vi "Synchronized AO Generation.vi"() -> ()   [LabVIEW 2018, in "GettingStarted_5785_Host.lvlib"]
uses:
  GettingStarted_5785_Host.lvlib
  <vilib>/userdefined/High Color/nirio_resource_hc.ctl
  <instrlib>/FlexRIO/API/Host/v1/NI FlexRIO/API/Get Property Reference - Fpga Small.vi
  <instrlib>/FlexRIO/API/Host/v1/NI FlexRIO/API/Configure Digital Edge Start Trigger.vi
  <instrlib>/FlexRIO/API/Host/v1/NI FlexRIO/API/Read Stream 1D WDT.vi
  <vilib>/FPGAPlugInAG/Dynamic/niLvFpga_Close_Dynamic.vi
  <vilib>/rvi/interface/nirviCloseFPGA/nirviCloseFPGA.xnode
  <resource>/objmgr/niflexrioapiStream.rc
  <instrlib>/FlexRIO/API/Host/v1/NI FlexRIO API v1.lvlib
  <resource>/objmgr/niflexrioapi.rc
  <instrlib>/_niInstr/Streaming/v1/Host/niInstr Streaming v1 Host.lvlib
panel:
  in  "flexrio tranceivers":T2(array[cluster])
  in  "amplitude":dbl=0.2 format="%0.2p"
  in  "sampling info":cluster{"Fs":dbl, "#s":dbl}={"Fs"=3200000000.0, "#s"=1600.0} {"Fs" format="%#_6p"}
  in  "frequency":dbl=32000000.0 format="%0.2p"
  out "read data":waveform(dbl)[](graph)
  in  "num samples":u64=65536
  out "generation active":bool[](array[boolean])
  in  "stop":bool
  in  "trigger source":string(combo)
  in  "trigger mode":enum16{"Immediate", "Digital"}(ring)
  out "error out":errorcluster
  # "This example demonstrates how to synchronize AO streams across multiple transceivers.\n\nThe same waveform is downloaded to each each device, and generation will begin on AO0 and AO1 when the start trigger is received.\n\nChannels AI0 and AI1 on the first device are continually acquired and displayed.\n\nThe suggested cable configuration is to loopback AO0 to AI0 on the first device, and connect AO0 from the second device to AI1 on the first device."
  # "Generation trigger configuration"
  # "Digital Trigger configuration"
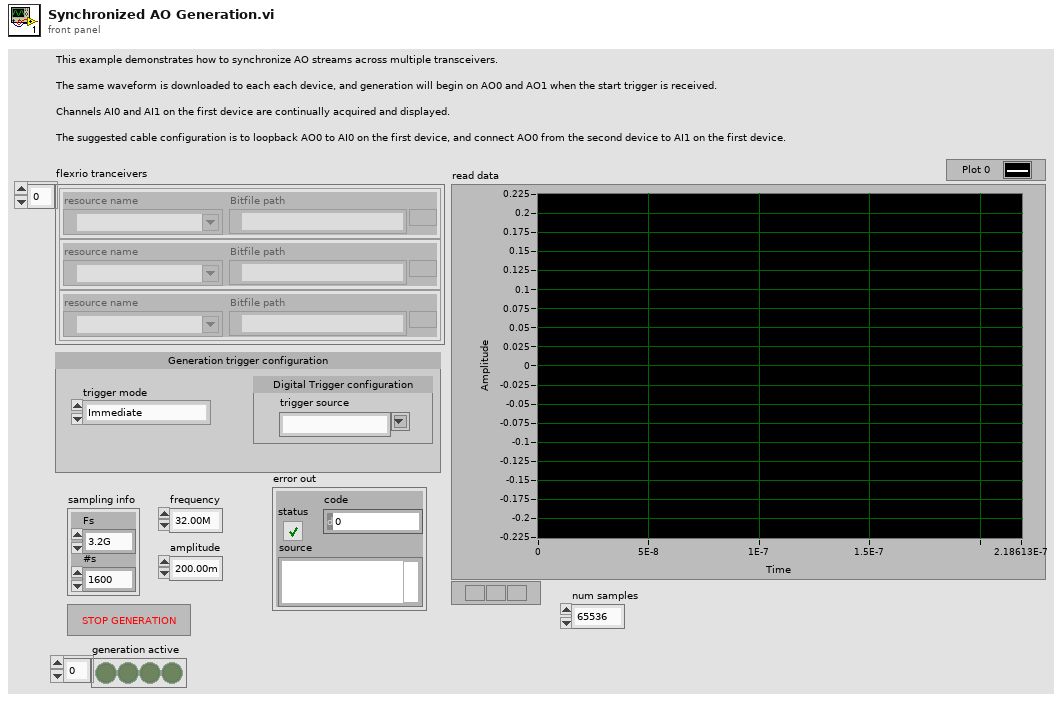
[diagram p1: front panel]
types:
  T1 = typedef "nirio_resource_hc.ctl" = tag
  T2 = cluster{"resource name":T1, "Bitfile path":path}[]
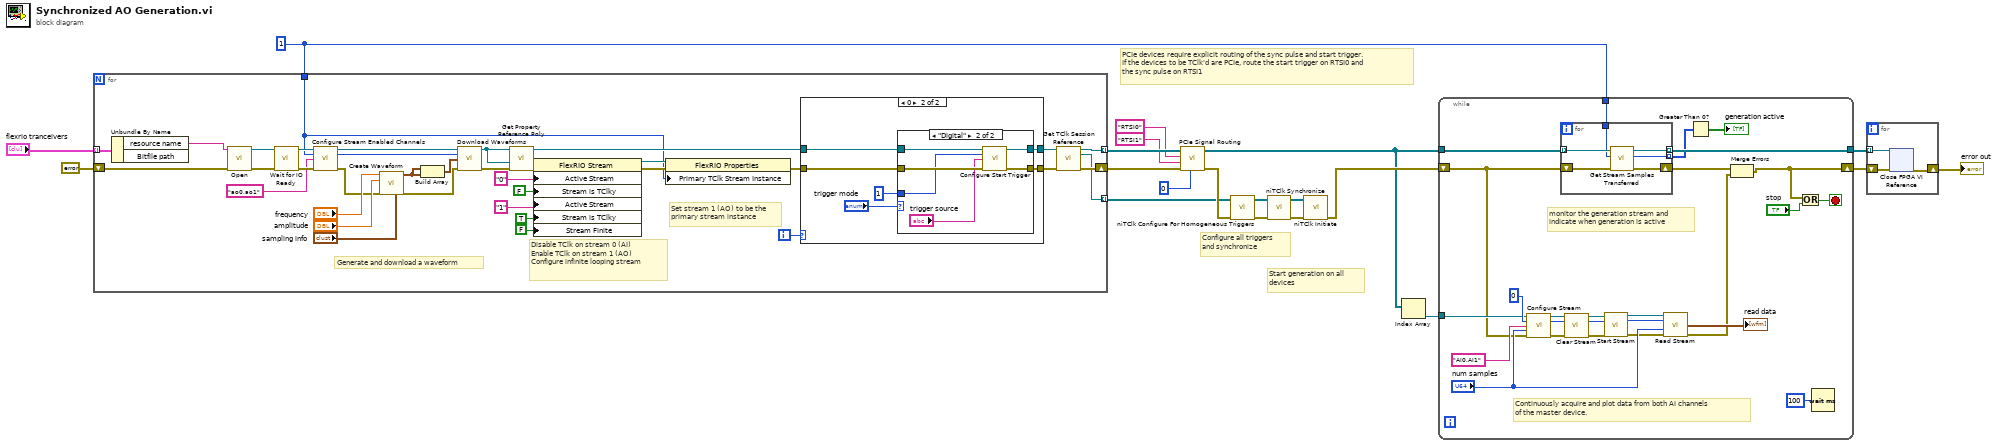
[diagram p0: block diagram]
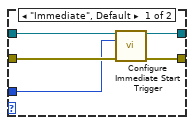
[diagram p3: hidden frame]
diagram:
  w3 = u32 1 ("stream instance")
  # "PCIe devices require explicit routing of the sync pulse and start trigger.\nIf the devices to be TClk'd are PCIe, route the start trigger on RTSI0 and\nthe sync pulse on RTSI1"
  # "Configure all triggers \nand synchronize"
  # "Start generation on all devices"
  n1 = for {
    tunnel: "flexrio tranceivers" -> [w40] mode=indexing
    tunnel: [w33] -> w7 mode=indexing
    shift-right: [w32] -> w9
    shift-left: errorcluster {"status"=FALSE, "code"=0, "source"=""} ("error out") -> [w48]
    tunnel: [w31] -> w6 mode=indexing
    tunnel: w3 -> [w23]
    i -> [w29]
    # "Set stream 1 (AO) to be the\nprimary stream instance"
    # "Disable TClk on stream 0 (AI)\nEnable TClk on stream 1 (AO)\nConfigure infinite looping stream"
    # "Generate and download a waveform"
    n2 = Unbundle By Name(w40) -> ("resource name"=w39:T1)  [unwired: 1 out]
    n3 = call <instrlib>:"Open.vi"("RIO Device"=w39, "error in"=w48) -> ("fpga interface out"=w37:refnum<k20>, "error out"=w38:errorcluster)  [unwired: 12 in]
    n4 = call <instrlib>:"Wait for IO Ready.vi"("fpga interface in"=w37, "error in"=w38) -> ("fpga interface out"=w27:refnum<k20>, "error out"=w26:errorcluster)  [unwired: 10 in, 2 out]
    n5 = call <instrlib>:"Configure Stream Enabled Channels.vi"("fpga interface in"=w27, "stream instance"=w23, "channels enabled"="ao0,ao1", "error in"=w26) -> ("fpga interface out"=w25:refnum<k20>, "stream instance out"=w22:u32, "error out"=w24:errorcluster)  [unwired: 8 in, 1 out]
    n6 = call "Create Waveform.vi"("sampling info"="sampling info", "error in (no error)"=w24, "amplitude"="amplitude", "frequency"="frequency") -> ("error out"=w46:errorcluster, "Output Waveform (V)"=w47:waveform(dbl))  [unwired: 5 in, 1 out]
    n7 = Build Array(w47, w47) -> (w45:waveform(dbl)[])
    n8 = call "Download Waveforms.vi"("fpga interface in"=w25, "stream instance"=w22, "waveforms"=w45, "error in"=w46) -> ("fpga interface out"=w36:refnum<k20>, "error out"=w44:errorcluster)  [unwired: 9 in, 1 out]
    n9 = call-poly <instrlib>:"Get Property Reference Poly.vi"("error in (no error)"=w44, "fpga interface in"=w36) -> ("error out"=w56:errorcluster, "property reference"=w55:refnum<k20>)  [unwired: 4 in, 1 out]
    n10 = property class="FlexRIO Stream"(reference=w55, error in=w56, "Active Stream"="0", "Stream is TClky"=FALSE ("Configuration:Stream is TClky"), "Active Stream"="1", "Stream is TClky"=TRUE ("Configuration:Stream is TClky"), "Stream Finite"=FALSE ("Configuration:Finite")) -> (reference out=w50:refnum<k20>, error out=w49:errorcluster)
    n11 = property class="FlexRIO Properties"(reference=w50, error in=w49, "Primary TClk Stream Instance"=w23) -> (error out=w30:errorcluster)  [unwired: 1 out]
    n12 = case shown="0" w29 {
      tunnel: w36 -> [w58 w62]
      tunnel: [w58 w61] -> w35
      tunnel: [w57 w60] -> w34
      tunnel: w30 -> [w57 w59]
      frame 1, Default {
      }
      frame 0 {
        n13 = case shown="\"Digital\"" "trigger mode" {
          tunnel: w59 -> [w69 w74]
          tunnel: w62 -> [w66 w75]
          tunnel: [w68 w73] -> w60
          tunnel: [w65 w72] -> w61
          tunnel: u32 1 ("trigger instance") -> [w67 w70]
          frame "Immediate", Default {
            n14 = call <instrlib>:"Configure Immediate Start Trigger.vi"("fpga interface in"=w66, "trigger instance"=w67, "error in"=w69) -> ("fpga interface out"=w65:refnum<k20>, "error out"=w68:errorcluster)  [unwired: 10 in, 1 out]
          }
          frame "Digital" {
            n15 = call-poly <instrlib>:"Configure Start Trigger.vi"("fpga interface in"=w75, "trigger instance"=w70, "trigger source"="trigger source", "error in"=w74) -> ("fpga interface out"=w72:refnum<k20>, "error out"=w73:errorcluster)  [unwired: 9 in, 1 out]
          }
        }
      }
    }
    n16 = call <instrlib>:"Get TClk Session Reference.vi"("fpga interface in"=w35, "error in"=w34) -> ("fpga interface out"=w33:refnum<k20>, "tclk session reference"=w31:refnum<k20>, "error out"=w32:errorcluster)  [unwired: 11 in]
  }
  n17 = call "PCIe Signal Routing.vi"("trigger master index"=0, "error in"=w9, "sync pulse rtsi line"="RTSI1", "start trigger rtsi line"="RTSI0", "fpga interfaces in"=w7) -> ("error out"=w8:errorcluster, "fpga interfaces out"=w1:refnum<k20>[])  [unwired: 5 in]
  n18 = call <instrlib>:"niTClk Configure For Homogeneous Triggers.vi"("error in (no error)"=w8, "sessions"=w6) -> ("error out"=w20:errorcluster, "sessions out"=w19:refnum<k20>[])  [unwired: 8 in]
  n19 = call <instrlib>:"niTClk Synchronize.vi"("error in (no error)"=w20, "sessions"=w19) -> ("error out"=w16:errorcluster, "sessions out"=w2:refnum<k20>[])  [unwired: 8 in]
  n20 = call <instrlib>:"niTClk Initiate.vi"("error in (no error)"=w16, "sessions"=w2) -> ("error out"=w15:errorcluster)  [unwired: 8 in, 1 out]
  n21 = Index Array(array=w1) -> (element=w14:refnum<k20>)  [unwired: 1 in]
  n22 = while {
    tunnel: w1 -> [w99]
    tunnel: [w98] -> w17
    tunnel: w14 -> [w81]
    shift-right: [w79] -> w13
    shift-left: w15 -> [w80]
    tunnel: w3 -> [w76]
    stop <- w101 stop-if-true
    # "Continuously acquire and plot data from both AI channels\nof the master device."
    # "monitor the generation stream and \nindicate when generation is active"
    n23 = call <instrlib>:"Configure Stream.vi"("fpga interface in"=w81, "stream instance"=u32 0, "channels enabled"="AI0,AI1", "num samples"="num samples", "error in"=w80) -> ("fpga interface out"=w92:refnum<k20>, "stream instance out"=w91:u32, "error out"=w90:errorcluster)  [unwired: 7 in, 1 out]
    n24 = for {
      shift-right: [w107] -> w78
      shift-left: w80 -> [w106]
      tunnel: w99 -> [w105] mode=indexing
      tunnel: [w104] -> w98 mode=indexing
      tunnel: [w103] -> w96 mode=indexing
      tunnel: w76 -> [w102]
      n25 = call <instrlib>:"Get Stream Samples Transferred.vi"("error in (no error)"=w106, "stream index"=w102, "refnum in"=w105) -> ("error out"=w107:errorcluster, "samples transferred"=w103:u64, "refnum out"=w104:refnum<k20>)  [unwired: 6 in]
    }
    n26 = call <instrlib>:"Clear Stream.vi"("fpga interface in"=w92, "stream instance"=w91, "error in"=w90) -> ("fpga interface out"=w86:refnum<k20>, "stream instance out"=w88:u32, "error out"=w87:errorcluster)  [unwired: 10 in]
    n27 = call <instrlib>:"Start Stream.vi"("fpga interface in"=w86, "stream instance"=w88, "error in"=w87) -> ("fpga interface out"=w85:refnum<k20>, "stream instance out"=w84:u32, "error out"=w83:errorcluster)  [unwired: 10 in]
    n28 = call-poly <instrlib>:"Read Stream.vi"("fpga interface in"=w85, "stream instance"=w84, "samples"="num samples", "error in"=w83) -> ("read data"=→"read data":waveform(dbl)[], "error out"=w77:errorcluster)  [unwired: 7 in, 3 out]
    n29 = Greater Than 0?(x=w96) -> (x > 0?=→"generation active":bool[])
    n30 = Merge Errors(w78, w77) -> (w79:errorcluster)
    n31 = Or(x=w79, y="stop") -> (x .or. y?=w101:bool)
    n32 = Wait (ms)(milliseconds to wait=u32 100) -> ()  [unwired: 1 out]
  }
  n33 = for {
    tunnel: w17 -> [w109] mode=indexing
    shift-right: [w108] -> w18
    shift-left: w13 -> [w110]
    n34 = xnode "Close FPGA VI Reference"("FPGA VI Reference In"=w109, "error in"=w110) -> ("error out"=w108:errorcluster)
  }
  "error out" <- w18
